vi "Microsync test.vi"() -> ()   [LabVIEW 2023]
uses:
  <vilib>/Instr/_visa.llb/VISA Configure Serial Port (Instr).vi
panel:
  in  "Property value to set":u32
  in  "prop to set":T1(ring)
  out "Property value":string
  in  "property":T1(ring)
  out "error out":errorcluster
  in  "VISA resource name":refnum<visa-resource-name>="COM5"
  out "Startup Message":string
  in  "error in (no error)":errorcluster
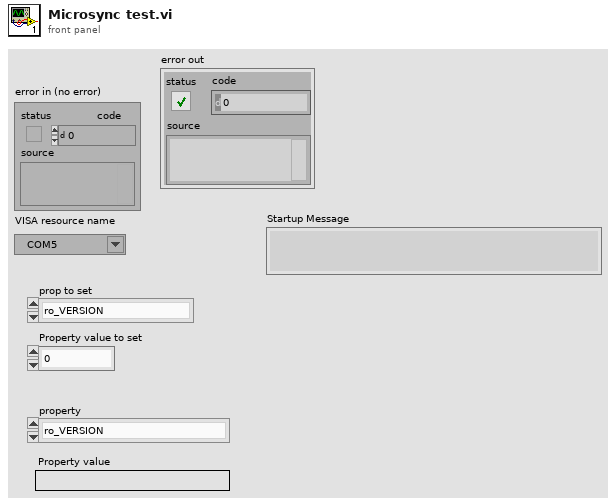
[diagram p1: front panel]
types:
  T1 = enum16{"ro_VERSION", "ro_SYS_TIMER_STATUS", "ro_SYS_TIMER_VALUE", "ro_SYS_TIMER_OVF_COUNT", "ro_SYS_TIME_ms", "ro_SYS_TIMER_PRESCALER", "rw_DFLT_PULSE_DURATION_us", "ro_WATCHDOG_TIMEOUT_ms", "ro_N_EVENTS", "rw_INTLCK_ENABLED", "rw_SELECTED_LASERS", "wo_OPEN_SHUTTERS", "wo_CLOSE_SHUTTERS", "rw_SHUTTER_DELAY_us", "rw_CAM_READOUT_us"}
  T2 = cluster{"interval_us":u32, "N":u32, "timestamp_us":u32, "arg2":u32, "arg1":u32}
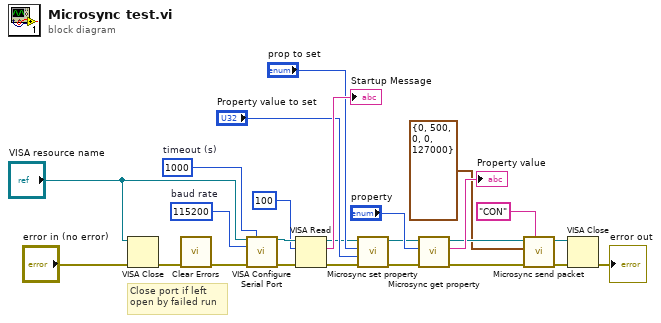
[diagram p0: block diagram]
diagram:
  w24 = u32 1000  # timeout (s)
  w25 = u32 115200  # baud rate
  # "Close port if left\nopen by failed run"
  n1 = VISA Close(VISA resource name="VISA resource name", error in (no error)="error in (no error)") -> (error out=w20:errorcluster)
  n2 = call <vilib>:"Clear Errors.vi"("error in (no error)"=w20) -> ("error out"=w19:errorcluster)  [unwired: 5 in, 1 out]
  n3 = call-poly "VISA Configure Serial Port"("VISA resource name"="VISA resource name", "timeout (10sec)"=w24, "baud rate (9600)"=w25, "error in (no error)"=w19) -> ("VISA resource name out"=w22:refnum<visa-resource-name>, "error out"=w23:errorcluster)  [unwired: 10 in]
  n4 = VISA Read(VISA resource name=w22, byte count=u32 100, error in (no error)=w23) -> (VISA resource name out=w5:refnum<visa-resource-name>, read buffer=→"Startup Message":string, error out=w4:errorcluster)  [unwired: 1 out]
  n5 = call "Microsync set property.vi"("error in (no error)"=w4, "Property value"="Property value to set", "property to set"="prop to set", "VISA resource name"=w5) -> ("error out"=w1:errorcluster, "VISA resource name out"=w2:refnum<visa-resource-name>)  [unwired: 6 in]
  n6 = call "Microsync get property.vi"("error in (no error)"=w1, "Property to get"="property", "VISA resource name"=w2) -> ("error out"=w11:errorcluster, "Retrieved property value"=→"Property value":string, "VISA resource name out"=w12:refnum<visa-resource-name>)  [unwired: 6 in]
  n7 = call "Microsync send packet.vi"("Command"="CON", "error in (no error)"=w11, "Arguments"=T2 {"interval_us"=0, "N"=500, "timestamp_us"=0, "arg2"=0, "arg1"=127000}, "VISA resource name"=w12) -> ("error out"=w10:errorcluster, "VISA resource name out"=w9:refnum<visa-resource-name>)  [unwired: 5 in, 1 out]
  n8 = VISA Close(VISA resource name=w9, error in (no error)=w10) -> (error out=→"error out":errorcluster)
